vi "REPORT_CFG_get_data_from_SQL.vi"(7 "type":T1 caption="Config:", 8 "error_in":errorcluster, 11 "dates_array":string[](array[string])) -> (0 "error_out":errorcluster, 3 "SQL_result":variant, 4 "executed_SQL_statement":string)   [LabVIEW 2020]
uses:
  typedef/REPORT_CFG_types.ctl
  FGV/SQL_connection/FGV_CLIENT_SQL_connection.ctl
  FGV/REPORTS_records_display/FGV_REPORTS_records_display.ctl
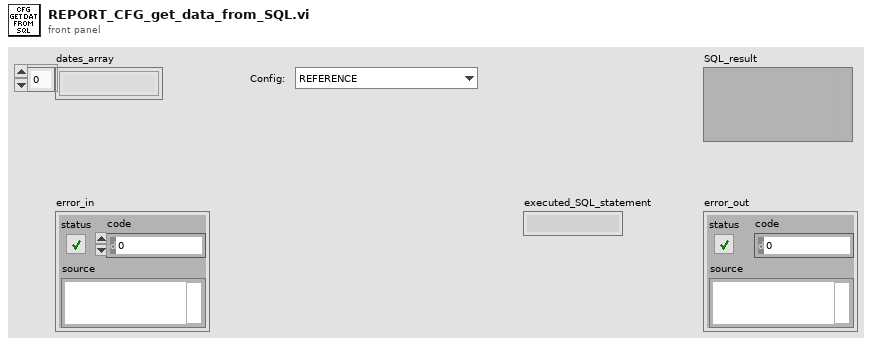
[diagram p1: front panel]
types:
  T1 = typedef "REPORT_CFG_types.ctl" = enum16{"REFERENCE", "ARCHIVISATION", "USERS", "ARCHIVISATION_AUDIT"}
  T2 = typedef "FGV_REPORTS_records_display.ctl" = enum16{"initialize", "GEAR_set_serial", "GEAR_set_header", "GEAR_set_operations", "GEAR_set_results", "GEAR_set_batches", "GEAR_get_serial", "GEAR_get_operation_IDs", "GEAR_toggle_results", "GEAR_show_all_results", "GEAR_hide_all_results", "GEAR_display", "GEAR_filter", "GEAR_restore", "GEAR_clear", "GEAR_get_all_info", "DATES_set_dates", "DATES_set_gears", "DATES_display", "DATES_filter", "DATES_first_page", "DATES_previous_page", "DATES_next_page", "DATES_last_page", "DATES_restore", "DATES_clear", "DATES_get_all_info", "PBATCH_set_batch_no", "PBATCH_set_gears", "PBATCH_display", "PBATCH_filter", "PBATCH_first_page", "PBATCH_previous_page", "PBATCH_next_page", "PBATCH_last_page", "PBATCH_restore", "PBATCH_clear", "PBATCH_get_all_info", "OPRTN_set_OP", "OPRTN_set_dates", "OPRTN_set_gears", "OPRTN_set_hidden_columns", "OPRTN_display", "OPRTN_filter", "OPRTN_filter_no_page_reset", "OPRTN_first_page", "OPRTN_previous_page", "OPRTN_next_page", "OPRTN_last_page", "OPRTN_restore", "OPRTN_clear", "OPRTN_get_all_info", "CFG_set_type", "CFG_set_dates", "CFG_set_records", "CFG_display", "CFG_filter", "CFG_first_page", "CFG_previous_page", "CFG_next_page", "CFG_last_page", "CFG_restore", "CFG_clear", "CFG_get_all_info", "AUDIT_set_dates", "AUDIT_set_records", "AUDIT_display", "AUDIT_filter", "AUDIT_first_page", "AUDIT_previous_page", "AUDIT_next_page", "AUDIT_last_page", "AUDIT_restore", "AUDIT_clear", "AUDIT_set_results", "AUDIT_get_all_info", "AUDIT_toggle_results", "AUDIT_show_all_results", "AUDIT_hide_all_results", "OKNOK_set_dates", "OKNOK_set_records", "OKNOK_display", "OKNOK_restore", "OKNOK_clear", "OKNOK_get_all_info", "REWORKS_set_dates", "REWORKS_set_from_to", "REWORKS_set_records", "REWORKS_display", "REWORKS_filter", "REWORKS_first_page", "REWORKS_previous_page", "REWORKS_next_page", "REWORKS_last_page", "REWORKS_restore", "REWORKS_clear", "REWORKS_get_all_info", "PACE_set_dates", "PACE_set_limits", "PACE_set_records", "PACE_display", "PACE_restore", "PACE_clear", "PACE_get_all_info", "CBATCH_set_code", "CBATCH_set_records", "CBATCH_display", "CBATCH_filter", "CBATCH_first_page", "CBATCH_previous_page", "CBATCH_next_page", "CBATCH_last_page", "CBATCH_restore", "CBATCH_clear", "CBATCH_get_all_info", "CMPNT_set_serial", "CMPNT_set_records", "CMPNT_display", "CMPNT_first_page", "CMPNT_previous_page", "CMPNT_next_page", "CMPNT_last_page", "CMPNT_restore", "CMPNT_clear", "CMPNT_get_all_info", "clear"}
  T3 = typedef "FGV_CLIENT_SQL_connection.ctl" = enum16{"initialize", "connect", "read_tables", "read_columns", "SELECT", "INSERT", "UPDATE", "DELETE", "EXEC + headers", "EXEC", "TRANSACTION", "connection_active?", "disconnect"}
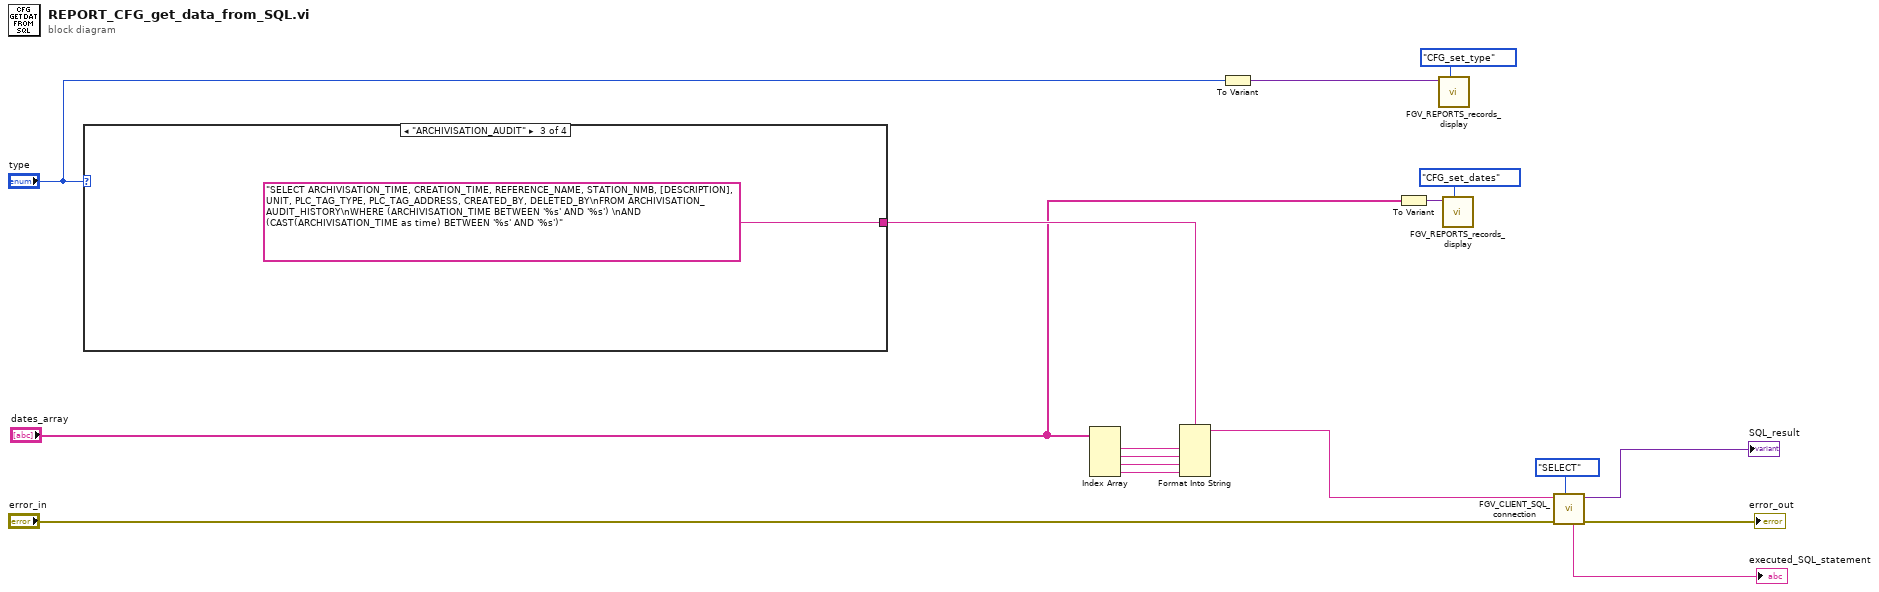
[diagram p0: block diagram]
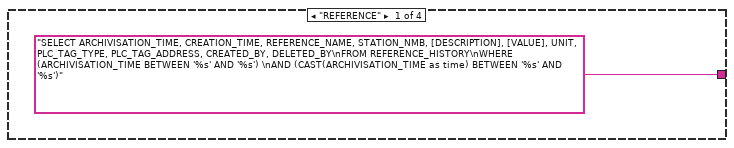
[diagram p2: hidden frame]
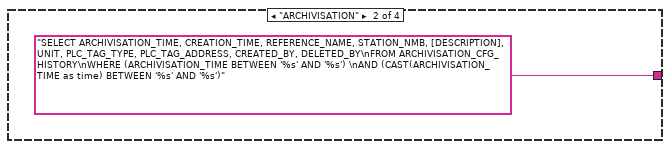
[diagram p3: hidden frame]
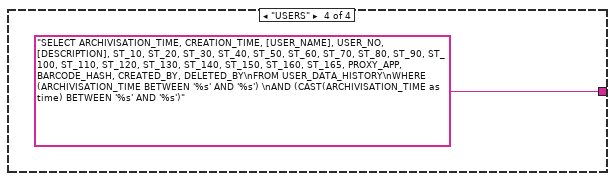
[diagram p4: hidden frame]
diagram:
  n1 = case shown="\"ARCHIVISATION_AUDIT\"" "type" {
    tunnel: ["SELECT ARCHIVISATION_TIME, CREATION_TIME, REFERENCE_NAME, STATION_NMB, [DESCRIPTION], [VALUE], UNIT, PLC_TAG_TYPE, PLC_TAG_ADDRESS, CREATED_BY, DELETED_BY\nFROM REFERENCE_HISTORY\nWHERE (ARCHIVISATION_TIME BETWEEN '%s' AND '%s') \nAND (CAST(ARCHIVISATION_TIME as time) BETWEEN '%s' AND '%s')" "SELECT ARCHIVISATION_TIME, CREATION_TIME, REFERENCE_NAME, STATION_NMB, [DESCRIPTION], UNIT, PLC_TAG_TYPE, PLC_TAG_ADDRESS, CREATED_BY, DELETED_BY\nFROM ARCHIVISATION_CFG_HISTORY\nWHERE (ARCHIVISATION_TIME BETWEEN '%s' AND '%s') \nAND (CAST(ARCHIVISATION_TIME as time) BETWEEN '%s' AND '%s')" "SELECT ARCHIVISATION_TIME, CREATION_TIME, REFERENCE_NAME, STATION_NMB, [DESCRIPTION], UNIT, PLC_TAG_TYPE, PLC_TAG_ADDRESS, CREATED_BY, DELETED_BY\nFROM ARCHIVISATION_AUDIT_HISTORY\nWHERE (ARCHIVISATION_TIME BETWEEN '%s' AND '%s') \nAND (CAST(ARCHIVISATION_TIME as time) BETWEEN '%s' AND '%s')" "SELECT ARCHIVISATION_TIME, CREATION_TIME, [USER_NAME], USER_NO, [DESCRIPTION], ST_10, ST_20, ST_30, ST_40, ST_50, ST_60, ST_70, ST_80, ST_90, ST_100, ST_110, ST_120, ST_130, ST_140, ST_150, ST_160, ST_165, PROXY_APP, BARCODE_HASH, CREATED_BY, DELETED_BY\nFROM USER_DATA_HISTORY\nWHERE (ARCHIVISATION_TIME BETWEEN '%s' AND '%s') \nAND (CAST(ARCHIVISATION_TIME as time) BETWEEN '%s' AND '%s')"] -> w4
    frame "REFERENCE" {
    }
    frame "ARCHIVISATION" {
    }
    frame "ARCHIVISATION_AUDIT" {
    }
    frame "USERS" {
    }
  }
  n2 = Index Array(array="dates_array") -> (element #1=w9:string, element #2=w8:string, element #3=w7:string, element #4=w6:string)  [unwired: 4 in]
  n3 = Format Into String(format string=w4, w9, w8, w7, w6) -> (resulting string=w13:string)  [unwired: 2 in, 1 out]
  n4 = To Variant(anything="type") -> (Variant=w10:variant)
  n5 = To Variant(anything="dates_array") -> (Variant=w2:variant)
  n6 = call "FGV_REPORTS_records_display.vi"("options"=FGV_REPORTS_records_display."CFG_set_type", "input"=w10) -> ()  [unwired: 8 in, 2 out]
  n7 = call "FGV_REPORTS_records_display.vi"("options"=FGV_REPORTS_records_display."CFG_set_dates", "input"=w2) -> ()  [unwired: 8 in, 2 out]
  n8 = call "FGV_CLIENT_SQL_connection.vi"("options"=FGV_CLIENT_SQL_connection."SELECT", "error_in"="error_in", "SQL_statement"=w13) -> ("error_out"=→"error_out":errorcluster, "SQL_result"=→"SQL_result":variant, "executed_SQL_statement"=→"executed_SQL_statement":string)  [unwired: 4 in, 2 out]
